vi "field raster.vi"(0 "field size":dbl, 2 "field number":dbl) -> (10 "Plot1":cluster{dbl[], dbl[]}, 11 "Plot2":cluster{dbl[], dbl[]}, 14 "current X":dbl, 15 "current Y":dbl, 17 "x mark":dbl[](array[numeric]), 18 "y mark":dbl[](array[numeric]))   [LabVIEW 2014]
uses:
  field-raster-globals.vi
panel:
  out "Xpseudo":dbl
  out "output variable 2":dbl
  out "output variable":dbl
  out "Ypseudo":dbl
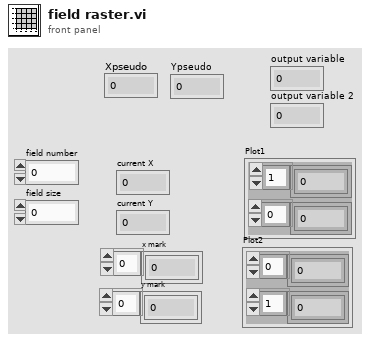
[diagram p1: front panel]
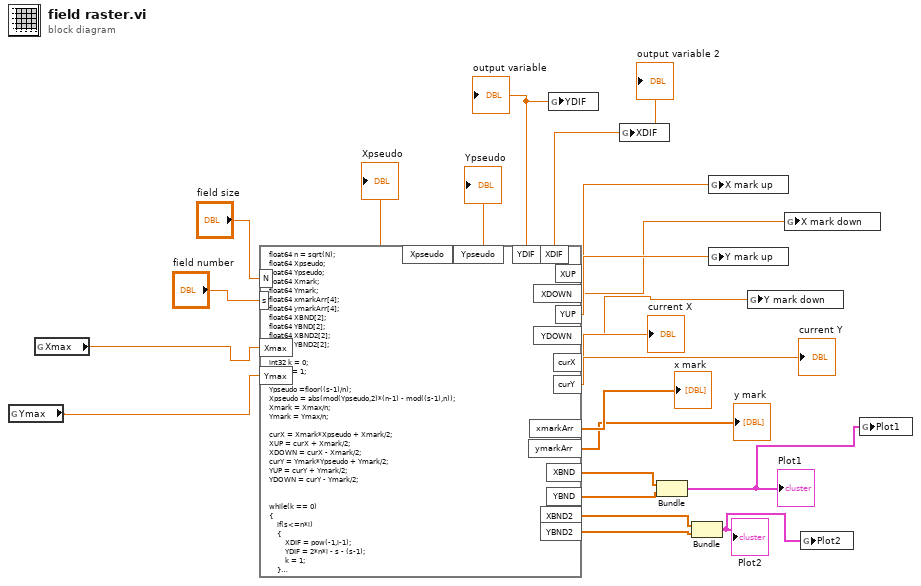
[diagram p0: block diagram]
diagram:
  n1 = global read "field-raster-globals.vi" "Ymax"() -> (w11:dbl)
  n2 = global read "field-raster-globals.vi" "Xmax"() -> (w12:dbl)
  n3 = formula code="float64 n = sqrt(N);\nfloat64 Xpseudo;\nfloat64 Ypseudo;\nfloat64 Xmark;\nfloat64 Ymark;\nfloat64 xmarkArr[4];\nfloat64 ymarkArr[4];\nfloat64 XBND[2];\nfloat64 YBND[2];\nfloat64 XBND2[2];\nfloat64 YBND2[2];\n\nint32 k = 0;\nint32 i = 1;\n\nYpseudo =floor((s-1)/n); \nXpseudo = abs(mod(Ypseudo,2)*(n-1) - mod((s-1),n));\nXmark = Xmax/n;\nYmark = Ymax/n;\n\ncurX = Xmark*Xpseudo + Xmark/2;\nXUP = curX + Xmark/2;\nXDOWN = curX - Xmark/2;\ncurY = Ymark*Ypseudo + Ymark/2;\nYUP = curY + Ymark/2;\nYDOWN = curY - Ymark/2;\n\n\nwhile(k == 0)\n{\n    if(s<=n*i)\n    {\n        XDIF = pow(-1,i-1);\n        YDIF = 2*n*i - s - (s-1);\n        k = 1;\n    }\n    i++;\n}\n\ni = 1;\n\nwhile(i < n)\n{\n   xmarkArr[i] = Xmark*i;\n   ymarkArr[i] = Ymark*i;\n   i++;\n}\n\ni = 0;\n\n XBND[i] = curX - Xmark/2;\nYBND[i] = curY - Ymark/2;\n i++;\nXBND[i] = curX + Xmark/2;\nYBND[i] = curY - Ymark/2;\n\ni=0;\n\nXBND2[i] = curX - Xmark/2;\nYBND2[i] =  curY + Ymark/2;\ni++;\nXBND2[i] = curX + Xmark/2;\nYBND2[i] =  curY + Ymark/2;\ni++;"("N"="field size", "s"="field number", "Xmax"=w12, "Ymax"=w11) -> ("curX"=→"current X":dbl, "curY"=→"current Y":dbl, "ymarkArr"=→"y mark":dbl[], "xmarkArr"=→"x mark":dbl[], "XUP"=w7:dbl, "YUP"=w8:dbl, "XBND"=w16:dbl[], "YBND"=w15:dbl[], "XBND2"=w14:dbl[], "YBND2"=w13:dbl[], "XDOWN"=w6:dbl, "YDOWN"=w5:dbl, "YDIF"=w4:dbl, "XDIF"=w3:dbl, "Ypseudo"=→"Ypseudo":dbl, "Xpseudo"=→"Xpseudo":dbl)
  "output variable" <- w4
  "output variable 2" <- w3
  n4 = global write "field-raster-globals.vi" "YDIF"(w4) -> ()
  n5 = global write "field-raster-globals.vi" "XDIF"(w3) -> ()
  n6 = Bundle(w16, w15) -> (w18:cluster{dbl[], dbl[]})  [unwired: 1 out]
  "Plot1" <- w18
  n7 = Bundle(w14, w13) -> (w17:cluster{dbl[], dbl[]})  [unwired: 1 out]
  "Plot2" <- w17
  n8 = global write "field-raster-globals.vi" "X mark up"(w7) -> ()
  n9 = global write "field-raster-globals.vi" "Y mark up"(w8) -> ()
  n10 = global write "field-raster-globals.vi" "Y mark down"(w5) -> ()
  n11 = global write "field-raster-globals.vi" "X mark down"(w6) -> ()
  n12 = global write "field-raster-globals.vi" "Plot2"(w17) -> ()
  n13 = global write "field-raster-globals.vi" "Plot1"(w18) -> ()
